vi "AWS IoT Button - Publish to SNS Topic.vi"() -> ()   [LabVIEW 2015]
doc: "Demonstrates how to programmatically publish AWS IoT Button data to an SNS topic."
uses:
  <vilib>/AWS Toolkit/Core/HTTP Request/Region.ctl
  <vilib>/AWS Toolkit/IoT/Topic Rule.ctl
  <vilib>/AWS Toolkit/IoT/CloudWatch Alarm.ctl
  <vilib>/AWS Toolkit/IoT/CloudWatch Metric.ctl
  <vilib>/AWS Toolkit/IoT/DynamoDB.ctl
  <vilib>/AWS Toolkit/IoT/DynamoDBv2.ctl
  <vilib>/AWS Toolkit/IoT/Elasticsearch.ctl
  <vilib>/AWS Toolkit/IoT/Firehose.ctl
  <vilib>/AWS Toolkit/IoT/Kinesis.ctl
  <vilib>/AWS Toolkit/IoT/Lambda.ctl
  <vilib>/AWS Toolkit/IoT/Republish.ctl
  <vilib>/AWS Toolkit/IoT/S3.ctl
  <vilib>/AWS Toolkit/IoT/SNS.ctl
  <vilib>/AWS Toolkit/IoT/SQS.ctl
  <vilib>/AWS Toolkit/SNS/Subscription/Subscription Protocol.ctl
  <vilib>/AWS Toolkit/Core/HTTP Request/AWS Credentials.ctl
  <vilib>/AWS Toolkit/Core/ARN/ARN.lvclass/ARN.ctl
  <vilib>/AWS Toolkit/Core/ARN/Read ARN.vi
  <vilib>/AWS Toolkit/IoT/IoT Session/IoT Session.lvclass
  <vilib>/AWS Toolkit/IoT/NI_AWS_IoT.lvlib
  <vilib>/AWS Toolkit/SNS/Topic/Topic.lvclass
  <vilib>/AWS Toolkit/SNS/Subscription/Subscription.lvclass
  <vilib>/AWS Toolkit/Core/HTTP Request/HTTP Request.lvclass
panel:
  in  "Email Address":string
  in  "SNS Topic Name":string
  in  "AWS IoT Button Serial Number":string
  in  "Region":T1
  in  "Secret Key":string
  in  "Access Key":string
  # "Overview: Demonstrates how to programmatically publish AWS IoT Button data to an SNS topic.\nRequirements: NI Cloud Toolkit for AWS, a configured AWS IoT Button, and a registered Amazon AWS account\nInstructions:\n1. Specify the Access Key and Secret Key for your AWS account. You can create an account at http://aws.amazon.com.\n2. Make sure you already have an AWS IoT Button configured in the AWS IoT Management Console on the amazon website.\n3. Specify the Region under which your AWS IoT Button is configured.\n4. Specify the AWS IoT Button Serial Number.\n5. Specify the SNS Topic Name where you want to publish the AWS IoT Button data. Note: This topic must already exist, and it must be in the same region as the AWS IoT Button.\n6. Specify the Email Address where you would like the SNS topic to publish the AWS IoT Button data.\n7. Run the VI.\n8. Click the 'Confirm Subscription' link in the email you should receive at the specified address.\n9. Click the AWS IoT Button. After the green light appears on the button, you should receive an email containing the AWS IoT Button data."
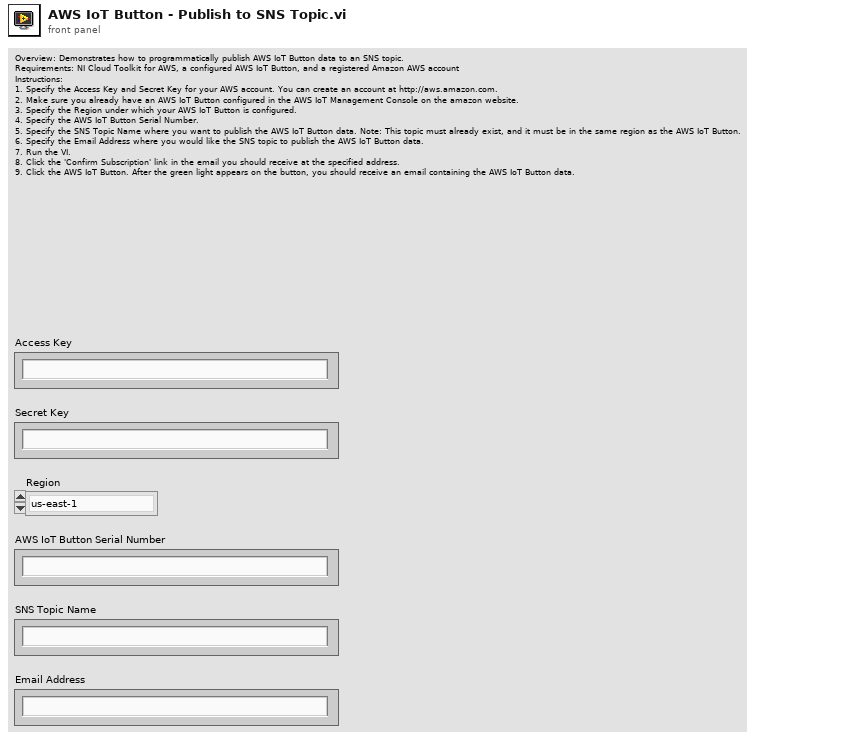
[diagram p1: front panel]
types:
  T1 = typedef "NI_AWS_Core.lvlib/HTTP Request.lvclass/Region.ctl" = enum16{"us-east-1", "us-east-2", "us-west-1", "us-west-2", "ap-northeast-1", "ap-northeast-2", "ap-southeast-1", "ap-southeast-2", "ca-central-1", "eu-central-1", "eu-west-1", "eu-west-2", "sa-east-1"}
  T2 = typedef "NI_AWS_Core.lvlib/HTTP Request.lvclass/AWS Credentials.ctl" = cluster{"Access Key":string, "Secret Key":string}
  T3 = typedef "NI_AWS_SNS.lvlib/Subscription.lvclass/Subscription Protocol.ctl" = enum16{"http", "https", "email", "email-json", "sms", "sqs", "application", "lambda"}
  T4 = typedef "NI_AWS_IoT.lvlib/SNS.ctl" = cluster{"Message Format":string, "Role ARN":string, "Target ARN":string}
  T5 = typedef "NI_AWS_IoT.lvlib/Topic Rule.ctl" = cluster{"CloudWatch Alarm":T6[], "CloudWatch Metric":T7[], "DynamoDB":T8[], "DynamoDBv2":T9[], "Elasticsearch":T10[], "Firehose":T11[], "Kinesis":T12[], "Lambda":T13[], "Republish":T14[], "S3":T15[], "SNS":T4[], "SQS":T16[], "AWS IoT SQL Version":string, "Description":string, "Created At":u64, "Incoming Schema ARN":string, "Outgoing Schema ARN":string, "Rule Disabled":bool, "Rule Name":string, "SQL":string, "Rule ARN":string}
  T6 = typedef "NI_AWS_IoT.lvlib/CloudWatch Alarm.ctl" = cluster{"Alarm Name":string, "Role ARN":string, "State Reason":string, "State Value":string}
  T7 = typedef "NI_AWS_IoT.lvlib/CloudWatch Metric.ctl" = cluster{"Metric Name":string, "Metric Namespace":string, "Metric Timestamp":string, "Metric Unit":string, "Metric Value":string, "Role ARN":string}
  T8 = typedef "NI_AWS_IoT.lvlib/DynamoDB.ctl" = cluster{"Hash Key Field":string, "Hash Key Type":string, "Hash Key Value":string, "Operation":string, "Payload Field":string, "Range Key Field":string, "Range Key Type":string, "Range Key Value":string, "Role ARN":string, "Table Name":string}
  T9 = typedef "NI_AWS_IoT.lvlib/DynamoDBv2.ctl" = cluster{"Role ARN":string, "Table Name":string}
  T10 = typedef "NI_AWS_IoT.lvlib/Elasticsearch.ctl" = cluster{"Endpoint":string, "ID":string, "Index":string, "Role ARN":string, "Type":string}
  T11 = typedef "NI_AWS_IoT.lvlib/Firehose.ctl" = cluster{"Delivery Stream Name":string, "Role ARN":string, "Separator":string}
  T12 = typedef "NI_AWS_IoT.lvlib/Kinesis.ctl" = cluster{"Partition Key":string, "Role ARN":string, "Stream Name":string}
  T13 = typedef "NI_AWS_IoT.lvlib/Lambda.ctl" = cluster{"Function ARN":string}
  T14 = typedef "NI_AWS_IoT.lvlib/Republish.ctl" = cluster{"Role ARN":string, "Topic":string}
  T15 = typedef "NI_AWS_IoT.lvlib/S3.ctl" = cluster{"Bucket Name":string, "Canned ACL":string, "Key":string, "Role ARN":string}
  T16 = typedef "NI_AWS_IoT.lvlib/SQS.ctl" = cluster{"Queue URL":string, "Role ARN":string, "Use Base 64":bool}
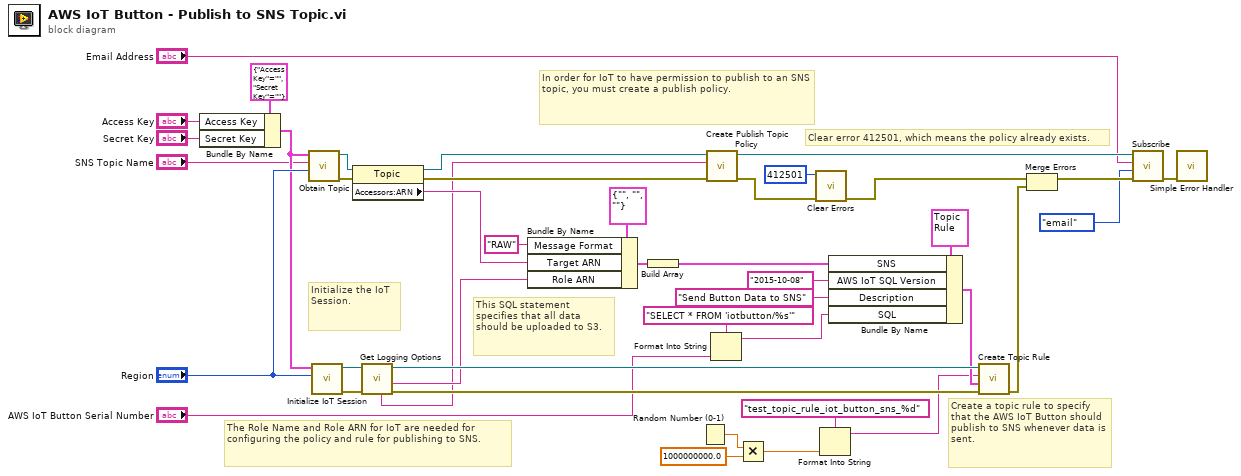
[diagram p0: block diagram]
diagram:
  # "This SQL statement specifies that all data should be uploaded to S3."
  # "Create a topic rule to specify that the AWS IoT Button should publish to SNS whenever data is sent."
  # "The Role Name and Role ARN for IoT are needed for configuring the policy and rule for publishing to SNS."
  # "Initialize the IoT Session."
  # "Clear error 412501, which means the policy already exists."
  # "In order for IoT to have permission to publish to an SNS topic, you must create a publish policy."
  n1 = Bundle By Name(cluster=T2 {"Access Key"="", "Secret Key"=""} ("AWS Credentials"), "Access Key"="Access Key", "Secret Key"="Secret Key") -> (w12:T2)
  n2 = call <vilib>:"Obtain Topic.vi"("Region"="Region", "Name"="SNS Topic Name", "AWS Credentials"=w12) -> ("error out"=w40:errorcluster, "Topic out"=w39:refnum<class "Topic.lvclass">)  [unwired: 7 in]
  n3 = call <vilib>:"Initialize IoT Session.vi"("Region"="Region", "AWS Credentials"=w12) -> ("error out"=w42:errorcluster, "IoT Session"=w36:refnum<class "IoT Session.lvclass">)  [unwired: 8 in]
  n4 = property class="Topic"(reference=w39, error in=w40) -> (reference out=w23:refnum<class "Topic.lvclass">, error out=w27:errorcluster, "Accessors:ARN"=w38:string)
  n5 = call <vilib>:"Get Logging Options.vi"("error in (no error)"=w42, "IoT Session in"=w36) -> ("error out"=w37:errorcluster, "Role ARN"=w34:string, "IoT Session out"=w35:refnum<class "IoT Session.lvclass">, "Role Name"=w22:string)  [unwired: 5 in, 1 out]
  n6 = Bundle By Name(cluster=T4 {"Message Format"="", "Role ARN"="", "Target ARN"=""} ("SNS"), "Message Format"="RAW", "Target ARN"=w38, "Role ARN"=w34) -> (w33:T4)
  n7 = Build Array(w33) -> (w21:T4[])
  n8 = Random Number (0-1)() -> (number: 0 to 1=w7:dbl)
  n9 = call <vilib>:"Create Publish Topic Policy.vi"("error in (no error)"=w27, "Role Name"=w22, "Topic in"=w23) -> ("error out"=w2:errorcluster, "Topic out"=w17:refnum<class "Topic.lvclass">)  [unwired: 7 in]
  n10 = Format Into String(format string="SELECT * FROM 'iotbutton/%s'", "AWS IoT Button Serial Number") -> (resulting string=w28:string)  [unwired: 2 in, 1 out]
  n11 = Multiply(x=w7, y=1000000000.0) -> (x*y=w5:dbl)
  n12 = call <vilib>:"Clear Errors.vi"("error in (no error)"=w2, "specific error code to clear (0: all)"=412501) -> ("error out"=w1:errorcluster)  [unwired: 4 in, 1 out]
  n13 = Format Into String(format string="test_topic_rule_iot_button_sns_%d" ("Name"), w5) -> (resulting string=w24:string)  [unwired: 2 in, 1 out]
  n14 = Bundle By Name(cluster=T5 {"CloudWatch Alarm"=[], "CloudWatch Metric"=[], "DynamoDB"=[], "DynamoDBv2"=[], "Elasticsearch"=[], "Firehose"=[], "Kinesis"=[], "Lambda"=[], "Republish"=[], "S3"=[], "SNS"=[], "SQS"=[], "AWS IoT SQL Version"="", "Description"="", "Created At"=0, "Incoming Schema ARN"="", "Outgoing Schema ARN"="", "Rule Disabled"=FALSE, "Rule Name"="", "SQL"="", "Rule ARN"=""} ("Topic Rule"), "SNS"=w21, "AWS IoT SQL Version"="2015-10-08", "Description"="Send Button Data to SNS", "SQL"=w28) -> (w30:T5)
  n15 = call <vilib>:"Create Topic Rule.vi"("error in (no error)"=w37, "Topic Rule"=w30, "Rule Name"=w24, "IoT Session in"=w35) -> ("error out"=w26:errorcluster)  [unwired: 6 in, 1 out]
  n16 = Merge Errors(w1, w26) -> (w18:errorcluster)
  n17 = call <vilib>:"Subscribe.vi"("error in (no error)"=w18, "Protocol"=Subscription_Protocol."email", "Endpoint"="Email Address", "Topic in"=w17) -> ("error out"=w4:errorcluster)  [unwired: 5 in, 2 out]
  n18 = call <vilib>:"Simple Error Handler.vi"("error in (no error)"=w4) -> ()  [unwired: 4 in, 5 out]
